vi "Deadband Joysticks.vi"(8 "Deadbands":dbl[](array[numeric]), 11 "Axes":dbl[](array[numeric])) -> (3 "Axes'":dbl[](array[numeric]))   [LabVIEW 2020]
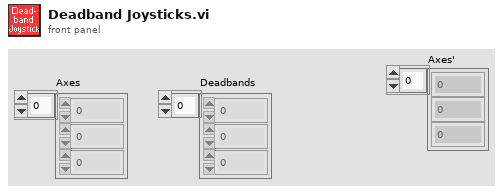
[diagram p1: front panel]
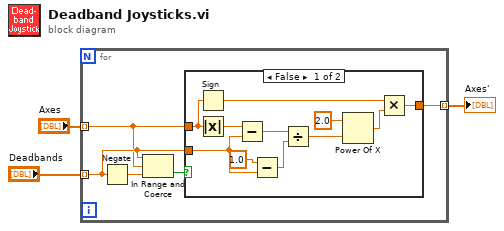
[diagram p0: block diagram]
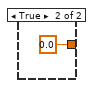
[diagram p2: hidden frame]
diagram:
  n1 = for {
    tunnel: "Deadbands" -> [w6] mode=indexing
    tunnel: "Axes" -> [w5] mode=indexing
    tunnel: [w4] -> w1 mode=indexing
    n2 = Negate(x=w6) -> (-x=w8:dbl)
    n3 = In Range and Coerce(upper limit=w6, x=w5, lower limit=w8) -> (In Range?=w7:bool)  [unwired: 1 out]
    n4 = case shown="False" w7 {
      tunnel: w6 -> [w14 _]
      tunnel: w5 -> [w13 _]
      tunnel: [w12 0.0] -> w4
      frame False {
        n5 = Sign(1:w13) -> (0:w15:dbl)
        n6 = Absolute Value(x=w13) -> (abs(x)=w18:dbl)
        n7 = Subtract(x=w18, y=w14) -> (x-y=w17:dbl)
        n8 = Subtract(x=1.0, y=w14) -> (x-y=w16:dbl)
        n9 = Divide(x=w17, y=w16) -> (x/y=w11:dbl)
        n10 = Power Of X(1:w11, 2:2.0 ("y")) -> (0:w9:dbl)
        n11 = Multiply(x=w15, y=w9) -> (x*y=w12:dbl)
      }
      frame True {
      }
    }
  }
  "Axes'" <- w1
